vi "Pre Launch Init.vi"(11 "Nested in":refnum<class "ImagePipeline.lvclass">) -> (0 "error out":errorcluster, 3 "Nested out":refnum<class "ImagePipeline.lvclass">)   [LabVIEW 2020, in "ImagePipeline.lvlib" / "ImagePipeline.lvclass"]
doc: "(<B>Filename</B>: Actor Framework.lvlib:Actor.lvclass:Pre Launch Init.vi)\n\nDefines behavior that occurs after the Launch Nested Actor method is invoked but before the actor's Actor Core method begins running.\n\nBy default, this method does nothing. A descendant class may override it to define behavior."
uses:
  ImagePipeline.lvclass
  ImagePipeline.lvclass/ImagePipeline.ctl
  <vilib>/ActorFramework/Actor/Actor.lvclass
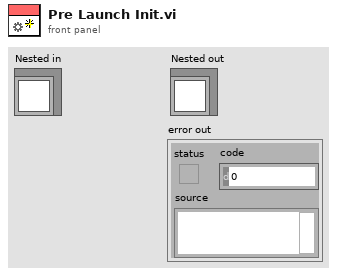
[diagram p1: front panel]
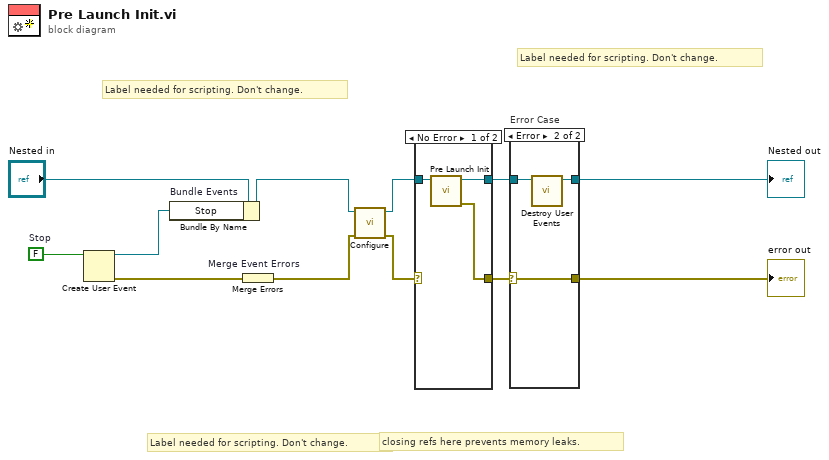
[diagram p0: block diagram]
diagram:
  w11 = FALSE  # Stop
  # "Label needed for scripting. Don't change."
  # "Label needed for scripting. Don't change."
  # "Label needed for scripting. Don't change."
  # "closing refs here prevents memory leaks."
  n1 = Create User Event(user event datatype=w11) -> (user event=w8:refnum<user-event>, error out=w10:errorcluster)  [unwired: 1 in]
  n2 = Bundle By Name "Bundle Events"(cluster="Nested in", "Stop"=w8) -> (w4:refnum<class "ImagePipeline.lvclass">)
  n3 = Merge Errors "Merge Event Errors"(w10) -> (w2:errorcluster)
  n4 = call-dynamic "Configure.vi"("error in (no error)"=w2, "ImagePipeline in"=w4) -> ("error out"=w1:errorcluster, "ImagePipeline out"=w3:refnum<class "ImagePipeline.lvclass">)  [unwired: 8 in]
  n5 = case shown="No Error" w1 {
    selector: w1 -> [_ w17]
    tunnel: [w15 w16] -> w6
    tunnel: w3 -> [w14 w16]
    tunnel: [w13 w17] -> w5
    frame No Error {
      n6 = call-parent "Pre Launch Init.vi"("Actor in"=w14) -> ("error out"=w13:errorcluster, "Actor out"=w15:refnum<class "ImagePipeline.lvclass">)  [unwired: 9 in]
    }
    frame Error {
    }
  }
  n7 = case "Error Case" shown="Error" w5 {
    selector: w5 -> [w18 w22]
    tunnel: w6 -> [w19 w21]
    tunnel: [w19 w20] -> w9
    tunnel: [w18 w22] -> w7
    frame No Error {
    }
    frame Error {
      n8 = call "Destroy User Events.vi"("UI Template in"=w21) -> ("UI Template out"=w20:refnum<class "ImagePipeline.lvclass">)  [unwired: 10 in]
    }
  }
  "error out" <- w7
  "Nested out" <- w9
